vi "Message and Response Example.vi"() -> ()   [LabVIEW 2011]
panel:
  in  "stop":bool
  in  "Send Message":bool
  in  "Message":string="hello"
  out "Response":string
  # "Message and Response Example\n\nPlease visit http://www.OpenG.org to learn about the\nOpen Source LabVIEW software movement.\n\nNOTICE -- YOU MUST LEAVE THIS NOTICE IN PLACE.  PER THE TERMS OF THE LICENSE BELOW, YOU MAY SUBLICENSE THIS SOFTWARE \nIN ANY WAY THAT DOES NOT CONFLICT WITH THIS LICENSE.\n\n### BSD License (http://www.opensource.org/licenses/bsd-license.php) Begin ###\n\nCopyright (c) 2008, Jim Kring <jim@jimkring.com>\nCopyright (c) 2010, Jonathon Green <jg@jgcode.net>\n\nAll rights reserved.\n\nRedistribution and use in source and binary forms, with or without modification, are permitted provided that the following conditions are met:\n\n    * Redistributions of source code must retain the above copyright notice, this list of conditions and the following disclaimer.\n    * Redistributions in binary form must reproduce the above copyright notice, this list of conditions and the following disclaimer in the \n       documentation and/or other materials provided with the distribution.\n    * Neither the name of SciWare, James Kring, Inc., nor the names of its contributors may be used to endorse or promote products derived \n       from this software without specific prior written permission.\n\nTHIS SOFTWARE IS PROVIDED BY THE COPYRIGHT HOLDERS AND CONTRIBUTORS \"AS IS\" AND ANY EXPRESS OR IMPLIED WARRANTIES, \nINCLUDING, BUT NOT LIMITED TO, THE IMPLIED WARRANTIES OF MERCHANTABILITY AND FITNESS FOR A PARTICULAR PURPOSE ARE \nDISCLAIMED. IN NO EVENT SHALL THE COPYRIGHT OWNER OR CONTRIBUTORS BE LIABLE FOR ANY DIRECT, INDIRECT, INCIDENTAL,\n SPECIAL, EXEMPLARY, OR CONSEQUENTIAL DAMAGES (INCLUDING, BUT NOT LIMITED TO, PROCUREMENT OF SUBSTITUTE GOODS OR \nSERVICES; LOSS OF USE, DATA, OR PROFITS; OR BUSINESS INTERRUPTION) HOWEVER CAUSED AND ON ANY THEORY OF LIABILITY, \nWHETHER IN CONTRACT, STRICT LIABILITY, OR TORT (INCLUDING NEGLIGENCE OR OTHERWISE) ARISING IN ANY WAY OUT OF THE USE \nOF THIS SOFTWARE, EVEN IF ADVISED OF THE POSSIBILITY OF SUCH DAMAGE.\n\n### BSD License End ###"
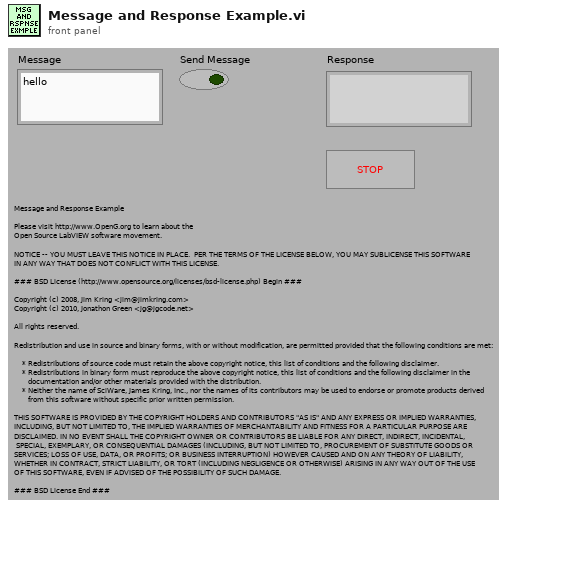
[diagram p1: front panel]
types:
  T1 = typedef "Msg Queue RefNum__ogtk.ctl" = refnum<k1>
  T2 = typedef "Notifier RefNum" = refnum<k1>
  T3 = typedef "Msg Cluster__ogtk.ctl" = cluster{"message":string, "response notifier":T2}
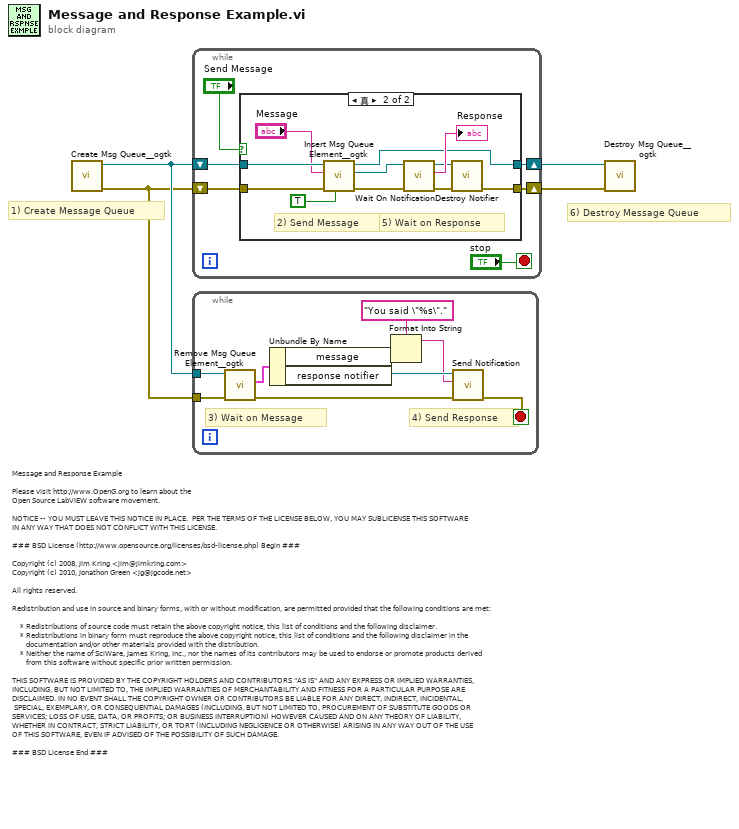
[diagram p0: block diagram]
diagram:
  # "Message and Response Example\n\nPlease visit http://www.OpenG.org to learn about the\nOpen Source LabVIEW software movement.\n\nNOTICE -- YOU MUST LEAVE THIS NOTICE IN PLACE.  PER THE TERMS OF THE LICENSE BELOW, YOU MAY SUBLICENSE THIS SOFTWARE \nIN ANY WAY THAT DOES NOT CONFLICT WITH THIS LICENSE.\n\n### BSD License (http://www.opensource.org/licenses/bsd-license.php) Begin ###\n\nCopyright (c) 2008, Jim Kring <jim@jimkring.com>\nCopyright (c) 2010, Jonathon Green <jg@jgcode.net>\n\nAll rights reserved.\n\nRedistribution and use in source and binary forms, with or without modification, are permitted provided that the following conditions are met:\n\n    * Redistributions of source code must retain the above copyright notice, this list of conditions and the following disclaimer.\n    * Redistributions in binary form must reproduce the above copyright notice, this list of conditions and the following disclaimer in the \n       documentation and/or other materials provided with the distribution.\n    * Neither the name of SciWare, James Kring, Inc., nor the names of its contributors may be used to endorse or promote products derived \n       from this software without specific prior written permission.\n\nTHIS SOFTWARE IS PROVIDED BY THE COPYRIGHT HOLDERS AND CONTRIBUTORS \"AS IS\" AND ANY EXPRESS OR IMPLIED WARRANTIES, \nINCLUDING, BUT NOT LIMITED TO, THE IMPLIED WARRANTIES OF MERCHANTABILITY AND FITNESS FOR A PARTICULAR PURPOSE ARE \nDISCLAIMED. IN NO EVENT SHALL THE COPYRIGHT OWNER OR CONTRIBUTORS BE LIABLE FOR ANY DIRECT, INDIRECT, INCIDENTAL,\n SPECIAL, EXEMPLARY, OR CONSEQUENTIAL DAMAGES (INCLUDING, BUT NOT LIMITED TO, PROCUREMENT OF SUBSTITUTE GOODS OR \nSERVICES; LOSS OF USE, DATA, OR PROFITS; OR BUSINESS INTERRUPTION) HOWEVER CAUSED AND ON ANY THEORY OF LIABILITY, \nWHETHER IN CONTRACT, STRICT LIABILITY, OR TORT (INCLUDING NEGLIGENCE OR OTHERWISE) ARISING IN ANY WAY OUT OF THE USE \nOF THIS SOFTWARE, EVEN IF ADVISED OF THE POSSIBILITY OF SUCH DAMAGE.\n\n### BSD License End ###"
  # "1) Create Message Queue"
  # "6) Destroy Message Queue"
  n1 = call <userlib>:"Create Msg Queue__ogtk.vi"() -> ("error out"=w1:errorcluster, "msg queue"=w2:T1)  [unwired: 5 in, 1 out]
  n2 = while {
    shift-right: [w7] -> w4
    shift-left: w1 -> [w9]
    shift-right: [w8] -> w3
    shift-left: w2 -> [w10]
    stop <- "stop" stop-if-true
    n3 = case shown="真" "Send Message" {
      tunnel: w10 -> [w12 w17]
      tunnel: w9 -> [w11 w18]
      tunnel: [w12 w16] -> w8
      tunnel: [w11 w20] -> w7
      frame False {
      }
      frame True {
        # "5) Wait on Response"
        # "2) Send Message"
        n4 = call <userlib>:"Insert Msg Queue Element__ogtk.vi"("Generate Response Notifier (F)"=TRUE, "error in (no error)"=w18, "message"="Message", "msg queue"=w17) -> ("error out"=w19:errorcluster, "response notifier"=w14:T2, "msg queue out"=w16:T1)  [unwired: 2 in, 1 out]
        n5 = call <vilib>:"Wait On Notification.vi"("error in (no error)"=w19, "notifier"=w14) -> ("error out"=w22:errorcluster, "notification"=→"Response":string, "notifier out"=w21:T2)  [unwired: 2 in, 1 out]
        n6 = call <vilib>:"Destroy Notifier.vi"("error in (no error)"=w22, "notifier"=w21) -> ("error out"=w20:errorcluster)  [unwired: 3 in, 2 out]
      }
    }
  }
  n7 = while {
    tunnel: w2 -> [w25]
    tunnel: w1 -> [w27]
    stop <- w28 stop-if-true
    # "4) Send Response"
    # "3) Wait on Message"
    n8 = call <userlib>:"Remove Msg Queue Element__ogtk.vi"("error in (no error)"=w27, "msg queue"=w25) -> ("error out"=w26:errorcluster, "message"=w24:T3)  [unwired: 6 in, 2 out]
    n9 = Unbundle By Name(w24) -> ("message"=w31:string, "response notifier"=w32:T2)
    n10 = Format Into String(format string="You said \"%s\".", w31) -> (resulting string=w29:string)  [unwired: 2 in, 1 out]
    n11 = call <vilib>:"Send Notification.vi"("error in (no error)"=w26, "notification"=w29, "notifier"=w32) -> ("error out"=w28:errorcluster)  [unwired: 3 in, 1 out]
  }
  n12 = call <userlib>:"Destroy Msg Queue__ogtk.vi"("error in (no error)"=w4, "msg queue"=w3) -> ()  [unwired: 3 in, 3 out]
